vi "Expt10 niUSRP EX QAM Tx student.vi"() -> ()   [LabVIEW 2024]
doc: "This example <B>requires the Modulation Toolkit</B>.\n\nApplies QAM (Quadrature Amplitude Modulation) to a PN sequence for USRP-based transmission. Continuously transmits a repeating message with a length determined by the PN Sequence Order parameter. \n\nThis example is paired with the example \"niUSRP Ex QAM Rx.vi\", which allows you to establish a Tx / Rx link between two separate USRPs. \n\nTo establish a Tx / Rx link between two USRPs:\n1) Ensure that the Tx and Rx example VIs have matching parameters for Modulation Scheme (M-Ary), Carrier Frequency, and Symbol Rate. Specify the Symbol Rate by setting the combination of the IQ Sampling Rate and the Number of Samples per Symbol parameters.\n2) Choose an IQ Sample Rate that enables sufficient Rx bandwidth.\n3) Set the Tx and / or Rx gain to ensure a sufficient signal to noise ratio on the Receive side. Note: applying too much gain can result in clipping.\n4) Choose a sufficient acquisition frame length that enables the demodulator to lock to the transmitted signal. National Instruments recommends that the acquired frame contain a number of symbols that is at least 20 * M-Ary of the modulation scheme. \n5) Ensure that the Reset Demodulator control is set to True until a solid lock is established. \n6) Install antennas and attenuators that efficiently operate at the carrier frequency you choose."
uses:
  <vilib>/addons/Modulation/niDMT.lvlib
  <instrlib>/niUSRP/niUSRP Write Tx Data (CDB Cluster).vi
panel:
  out "error out":errorcluster
  in  "Enabled Channel":string(combo)="0"
  out "Gain [dB] (actual)":dbl format="%#.6p"
  out "Carrier Frequency \n[Hz] (actual)":dbl=915000000.0 format="%#.6p"
  out "IQ Sampling\nRate [S/sec] (actual)":dbl=500000.0 format="%#.6p"
  in  "Active Antenna":string(combo)="TX1"
  in  "Gain [dB]":dbl format="%#.6p"
  in  "Carrier\nFrequency [Hz]":dbl=915000000.0 format="%#.6p"
  in  "IQ Sampling\nRate [S/sec]":dbl=500000.0 format="%#.6p"
  in  "Device Name":refnum<k15>="192.168.10.5"
  out "Frame Length [samples]":i32=2044
  in  "Pn Sequence Order":i32=13
  in  "Filter Parameters":T1={"Alpha"=0.5, "Filter Length"=6, "TX Filter"=enum."Root Raised Cos"} caption="Pulse Shaping Filter" {"Alpha" format="%.2f"}
  in  "QAM M-Ary":enum16{"4", "8", "16", "32", "64", "128", "256"}(ring)=enum."16"
  out "Symbol Rate [symbols/sec]":dbl=500000.0 format="%#.6p"
  in  "Samples Per Symbol":i32=4 min=2 step=2
  in  "Stop":bool
  out "Constellation Graph":T2(graph) caption="Tx Signal Constellation"
  # "Note:\nFrame size (samples per write) =\n (2^Pn Sequence Order) * Samples Per Symbol.\nUse Pn Sequence Order of 12 when using a 1 Gb Ethernet connection on a USRP RIO device. This prevents underflows by implicitly choosing \na frame size close to the ideal frame size for Ethernet connection. Refer to the \"Data Streaming Performance Tips\" section in the NI-USRP Help at ni.com/manuals for more information."
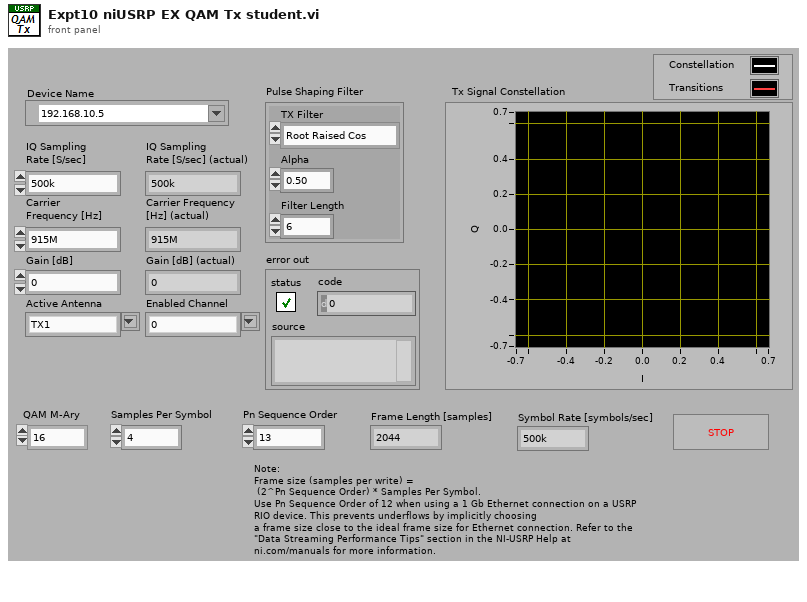
[diagram p1: front panel]
types:
  T1 = cluster{"Alpha":dbl, "Filter Length":i32, "TX Filter":enum16{"none", "Raised Cosine", "Root Raised Cos", "Gaussian"}}
  T2 = cluster{"constellation":dbl[], "oversampled data":dbl[]}[]
  T3 = enum32{"PN sequence", "User-defined pattern", "Read from file"}
  T4 = cluster{"samples per symbol (16)":i32, "symbol map":cdb[]}
  T5 = typedef "niAMT.lvlib/Complex Data Waveform.ctl" = cluster{"t0":dbl, "dt":dbl, "Y":cdb[]}
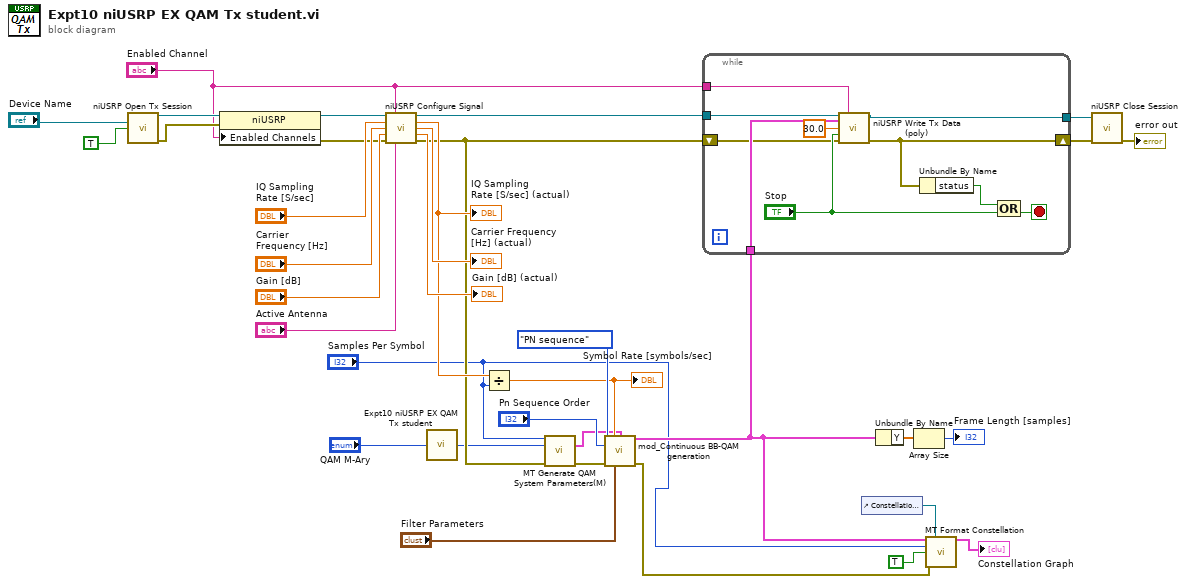
[diagram p0: block diagram]
diagram:
  n1 = call <instrlib>:"niUSRP Open Tx Session.vi"("device names"="Device Name", "reset"=TRUE) -> ("session handle out"=w17:refnum<k15>, "error out"=w15:errorcluster)  [unwired: 12 in]
  n2 = property class="niUSRP"(reference=w17, error in=w15, "Enabled Channels"="Enabled Channel") -> (reference out=w16:refnum<k15>, error out=w14:errorcluster)
  n3 = call <instrlib>:"niUSRP Configure Signal.vi"("session handle"=w16, "channel list"="Enabled Channel", "IQ rate"="IQ Sampling\nRate [S/sec]", "carrier frequency"="Carrier\nFrequency [Hz]", "gain"="Gain [dB]", "error in (no error)"=w14, "active antenna"="Active Antenna") -> ("session handle out"=w19:refnum<k15>, "coerced IQ rate"=w18:dbl, "coerced carrier frequency"=→"Carrier Frequency \n[Hz] (actual)":dbl, "coerced gain"=→"Gain [dB] (actual)":dbl, "error out"=w4:errorcluster)  [unwired: 4 in]
  "IQ Sampling\nRate [S/sec] (actual)" <- w18
  n4 = call "Expt10 niUSRP EX QAM Tx student.vi"("QAM M-ary"="QAM M-Ary") -> ("M-QAM"=w3:i32)
  n5 = Divide(x=w18, y="Samples Per Symbol") -> (x/y=w6:dbl)
  "Symbol Rate [symbols/sec]" <- w6
  n6 = call <vilib>:"MT Generate QAM System Parameters(M).vi"("samples per symbol (16)"="Samples Per Symbol", "M-QAM (16)"=w3, "error in (no error)"=w4) -> ("QAM system parameters"=w1:T4, "error out"=w5:errorcluster)  [unwired: 10 in, 1 out]
  n7 = call <vilib>:"mod_Continuous BB-QAM generation.vi"("Bit stream"=T3."PN sequence", "Symbol Rate, Hz"=w6, "QAM system parameters"=w1, "PN Sequence Order"="Pn Sequence Order", "error in (no error)"=w5, "filter parameters"="Filter Parameters") -> ("output complex waveform"=w7:T5, "error out"=w8:errorcluster)  [unwired: 5 in, 3 out]
  n8 = while {
    tunnel: [w43] -> w29
    tunnel: w19 -> [w45]
    shift-right: [w36] -> w28
    shift-left: w4 -> [w39]
    tunnel: w7 -> [w44]
    tunnel: "Enabled Channel" -> [w38]
    stop <- w40 stop-if-true
    n9 = call-poly <instrlib>:"niUSRP Write Tx Data (poly).vi"("session handle"=w45, "channel list"=w38, "data"=w44, "timeout"=30.0, "end of data?"="Stop", "error in (no error)"=w39) -> ("session handle out"=w43:refnum<k15>, "error out"=w36:errorcluster)  [unwired: 8 in]
    n10 = Unbundle By Name(w36) -> ("status"=w42:bool)
    n11 = Compound Arithmetic op=OR(w42, "Stop") -> (w40:bool)
  }
  n12 = control-ref of="Constellation Graph"() -> (w10:refnum<vi>)
  n13 = Unbundle By Name(w7) -> ("Y"=w35:cdb[])
  n14 = Array Size(array=w35) -> (size(s)=→"Frame Length [samples]":i32)
  n15 = call <vilib>:"MT Format Constellation.vi"("waveform"=w7, "constellation reference"=w10, "samples per symbol"="Samples Per Symbol", "autoscale"=TRUE, "error in (no error)"=w8) -> ("constellation graph"=→"Constellation Graph":T2)  [unwired: 9 in, 1 out]
  n16 = call <instrlib>:"niUSRP Close Session.vi"("session handle"=w29, "error in (no error)"=w28) -> ("error out"=→"error out":errorcluster)  [unwired: 13 in]
